vi "Arm PID.vi"(8 "Arm Down":bool, 9 "Arm Up":bool, 11 "Arm Setpoint":dbl) -> ()   [LabVIEW 2015]
uses:
  <vilib>/addons/control/pid/pid.llb/PID (DBL).vi
  <vilib>/addons/control/pid/NI_PID_pid.lvlib
panel:
  in  "PID gains":T1={"proportional gain (Kc)"=1.0, "integral time (Ti, min)"=0.01, "derivative time (Td, min)"=0.0} {"derivative time (Td, min)" format="%.3f"; "integral time (Ti, min)" format="%.3f"; "proportional gain (Kc)" format="%.3f"}
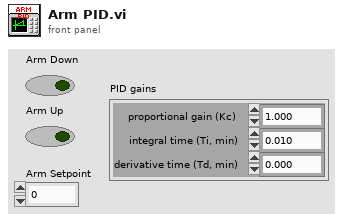
[diagram p1: front panel]
types:
  T1 = cluster{"proportional gain (Kc)":dbl, "integral time (Ti, min)":dbl, "derivative time (Td, min)":dbl}
  T2 = typedef "WPI_PotentiometerDevRef.ctl" = cluster{"DevStatus":errorcluster, "Analog Channel":T3, "Invert Output":bool}
  T3 = typedef "FPGA_AIChannel.ctl" = enum8{"AI 0", "AI 1", "AI 2", "AI 3", "AI MXP 0", "AI MXP 1", "AI MXP 2", "AI MXP 3", "Invalid"}
  T4 = typedef "WPI_MotorControlDeviceRef.ctl" = cluster{"DeviceStatus":errorcluster, "Type":T5, "PWM":cluster{"PWM Channel":T6, "DeadBand":T7}, "CAN":cluster{"Device Number":u8, "Control Mode":T8, "Semaphore":T9, "Max Vout":dbl, "TalonSRX Control Mode":T10}, "Invert":bool}
  T5 = typedef "WPI_MotorControlType.ctl" = enum16{"PWM", "CAN", "CANTalonSRX"}
  T6 = typedef "FPGA_DIOPWMChannel.ctl" = enum8{"PWM 0", "PWM 1", "PWM 2", "PWM 3", "PWM 4", "PWM 5", "PWM 6", "PWM 7", "PWM 8", "PWM 9", "PWM MXP 0", "PWM MXP 1", "PWM MXP 2", "PWM MXP 3", "PWM MXP 4", "PWM MXP 5", "PWM MXP 6", "PWM MXP 7", "PWM MXP 8", "PWM MXP 9", "Invalid"}
  T7 = typedef "WPI_PWMDeadband.ctl" = cluster{"Name":string, "maxPositivePwm":i32, "minPositivePwm":i32, "centerPwm":i32, "maxNegativePwm":i32, "minNegativePwm":i32, "angularRange":u16}
  T8 = typedef "WPI_CANJaguar_ControlMode.ctl" = enum8{"Percent VBus", "Current", "Speed", "Position", "Voltage"}
  T9 = typedef "Semaphore RefNum" = refnum<k1>
  T10 = typedef "WPI_CANTalonSRX_APIControlMode.ctl" = enum8{"Percent VBus", "Speed", "Position", "Slave", "Unchanged / Invalid", "Voltage Compensation", "Current", "Motion Profile"}
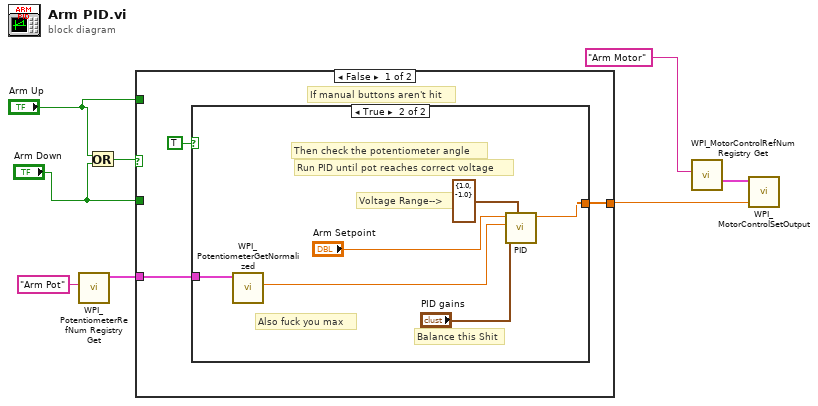
[diagram p0: block diagram]
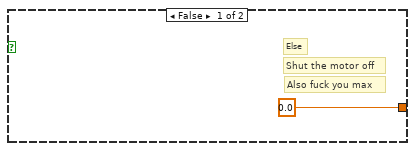
[diagram p2: hidden frame]
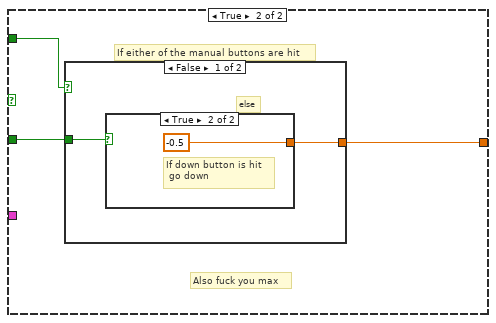
[diagram p3: hidden frame]
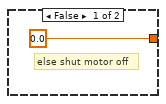
[diagram p4: hidden frame]
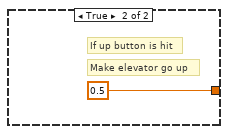
[diagram p5: hidden frame]
diagram:
  n1 = call <vilib>:"WPI_PotentiometerRefNum Registry Get.vi"("refnum name"="Arm Pot") -> ("PotDevRef"=w5:T2)  [unwired: 9 in, 1 out]
  n2 = Or(x="Arm Up", y="Arm Down") -> (x .or. y?=w3:bool)
  n3 = case shown="False" w3 {
    tunnel: [w11 w21] -> w8
    tunnel: w5 -> [w10 _]
    tunnel: "Arm Down" -> [_ w20]
    tunnel: "Arm Up" -> [_ w19]
    frame False {
      # "If manual buttons aren't hit"
      n4 = case shown="True" TRUE {
        tunnel: [0.0 w18] -> w11
        tunnel: w10 -> [_ w14]
        frame False {
          # "Also fuck you max"
          # "Shut the motor off"
          # "Else"
        }
        frame True {
          # "Voltage Range-->"
          # "Also fuck you max"
          # "Run PID until pot reaches correct voltage"
          # "Then check the potentiometer angle"
          # "Balance this Shit"
          n5 = call <vilib>:"WPI_PotentiometerGetNormalized.vi"("PotDevRef"=w14) -> ("Normalized Value"=w16:dbl)  [unwired: 8 in, 2 out]
          n6 = call-poly <vilib>:"PID.vi"("output range"=cluster{"output high":dbl, "output low":dbl} {"output high"=1.0, "output low"=-1.0}, "PID gains"="PID gains", "process variable"=w16, "setpoint"="Arm Setpoint") -> ("output"=w18:dbl)  [unwired: 6 in, 1 out]
        }
      }
    }
    frame True {
      # "Also fuck you max"
      # "If either of the manual buttons are hit"
      n7 = case shown="False" w19 {
        tunnel: [w23 0.5] -> w21
        tunnel: w20 -> [w22 _]
        frame False {
          # "else"
          n8 = case shown="True" w22 {
            tunnel: [0.0 -0.5] -> w23
            frame False {
              # "else shut motor off"
            }
            frame True {
              # "If down button is hit\n go down"
            }
          }
        }
        frame True {
          # "Make elevator go up"
          # "If up button is hit"
        }
      }
    }
  }
  n9 = call <vilib>:"WPI_MotorControlRefNum Registry Get.vi"("refnum name"="Arm Motor") -> ("MotorControlDevRef"=w7:T4)  [unwired: 9 in, 1 out]
  n10 = call <vilib>:"WPI_MotorControlSetOutput.vi"("Output"=w8, "MotorControlDevRef"=w7) -> ()  [unwired: 7 in, 3 out]
